vi "victor_linearize.vi"(11 "Input":dbl) -> (3 "Output":dbl)   [LabVIEW 2011]
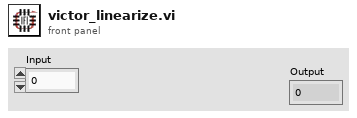
[diagram p1: front panel]
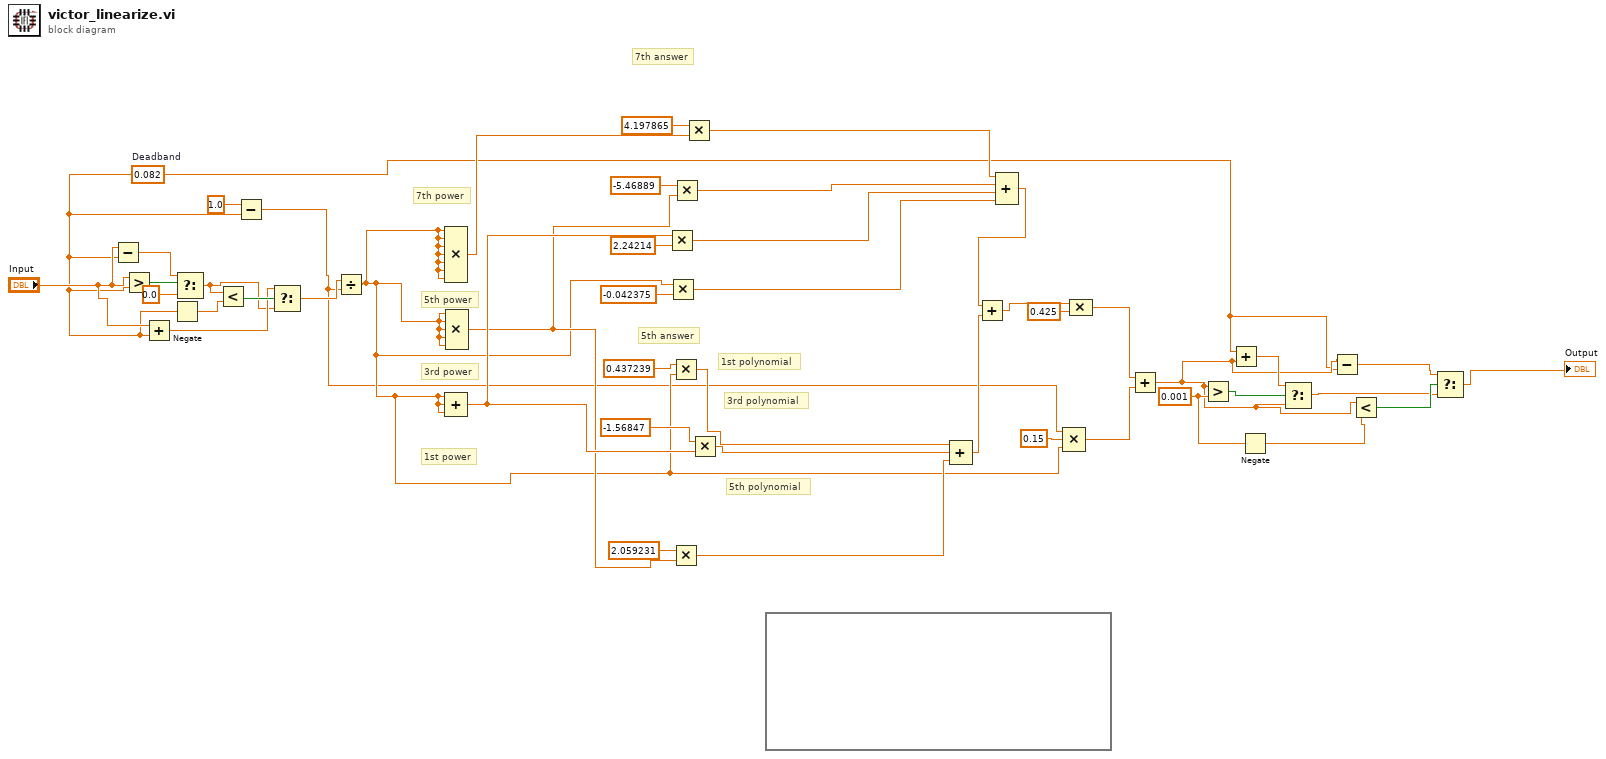
[diagram p0: block diagram]
diagram:
  w8 = 0.001 ("y")
  w3 = 0.082  # Deadband
  # "5th polynomial"
  # "3rd polynomial"
  # "1st polynomial"
  # "5th answer"
  # "7th answer"
  # "3rd power"
  # "1st power"
  # "5th power"
  # "7th power"
  n1 = Subtract(x="Input", y=w3) -> (x-y=w20:dbl)
  n2 = Greater?(x="Input", y=w3) -> (0:w21:bool)
  n3 = Add(x="Input", y=w3) -> (x+y=w16:dbl)
  n4 = Negate(x=w3) -> (-x=w18:dbl)
  n5 = Select(t=w20, s=w21, f=0.0) -> (s? t:f=w15:dbl)
  n6 = Less?(x=w15, y=w18) -> (x < y?=w17:bool)
  n7 = Subtract(x=1.0, y=w3) -> (x-y=w12:dbl)
  n8 = Select(t=w16, s=w17, f=w15) -> (s? t:f=w13:dbl)
  n9 = Divide(x=w13, y=w12) -> (x/y=w14:dbl)
  n10 = Compound Arithmetic op=MULTIPLY(w14, w14, w14, w14, w14, w14, w14) -> (w33:dbl)
  n11 = Compound Arithmetic op=ADD(w14, w14, w14) -> (w41:dbl)
  n12 = Compound Arithmetic op=MULTIPLY(w14, w14, w14, w14, w14) -> (w40:dbl)
  n13 = Multiply(x=w41, y=2.24214) -> (x*y=w38:dbl)
  n14 = Multiply(x=w14, y=-0.042375) -> (x*y=w39:dbl)
  n15 = Multiply(x=0.437239, y=w14) -> (x*y=w44:dbl)
  n16 = Multiply(x=2.059231, y=w40) -> (x*y=w42:dbl)
  n17 = Multiply(x=-5.46889, y=w40) -> (x*y=w37:dbl)
  n18 = Multiply(x=4.197865, y=w33) -> (x*y=w32:dbl)
  n19 = Multiply(x=-1.56847, y=w41) -> (x*y=w43:dbl)
  n20 = formula code=""() -> ()
  n21 = Compound Arithmetic op=ADD(w44, w43, w42) -> (w30:dbl)
  n22 = Compound Arithmetic op=ADD(w32, w37, w38, w39) -> (w31:dbl)
  n23 = Add(x=w31, y=w30) -> (x+y=w26:dbl)
  n24 = Compound Arithmetic op=MULTIPLY(w12, 0.15 ("x"), w14) -> (w28:dbl)
  n25 = Compound Arithmetic op=MULTIPLY(w26, 0.425 ("value")) -> (w27:dbl)
  n26 = Add(x=w27, y=w28) -> (x+y=w4:dbl)
  n27 = Greater?(x=w4, y=w8) -> (0:w9:bool)
  n28 = Add(x=w3, y=w4) -> (x+y=w10:dbl)
  n29 = Negate(x=w8) -> (-x=w7:dbl)
  n30 = Select(t=w10, s=w9, f=w4) -> (s? t:f=w5:dbl)
  n31 = Subtract(x=w4, y=w3) -> (x-y=w2:dbl)
  n32 = Less?(x=w4, y=w7) -> (x < y?=w6:bool)
  n33 = Select(t=w2, s=w6, f=w5) -> (s? t:f=→"Output":dbl)
